vi "监控模板.vi"() -> ()   [LabVIEW 2011]
panel:
  in  "监控":enum32{"RF", "TIME"}(tab)
  out "b 1":bool
  out "b 2":bool
  out "b 3":bool
  out "b 4":bool
  out "b 5":bool
  out "b 6":bool
  out "b 7":bool
  out "b 8":bool
  out "b 9":bool
  out "b 10":bool
  out "b 11":bool
  out "b 12":bool
  out "b 13":bool
  out "b 14":bool
  out "b 15":bool
  out "b 16":bool
  out "b 17":bool
  out "b 18":bool
  out "b 19":bool
  out "b 20":bool
  out "b 21":bool
  out "b 22":bool
  out "b 23":bool
  out "b 24":bool
  out "b 25":bool
  out "b 26":bool
  out "b 27":bool
  out "b 28":bool
  out "b 29":bool
  out "b 30":bool
  out "b 31":bool
  out "b 32":bool
  out "S 1":string
  out "S 2":string
  out "S 3":string
  out "S 4":string
  out "S 5":string
  out "S 6":string
  out "S 7":string
  out "S 8":string
  out "S 9":string
  out "S 10":string
  out "S 11":string
  out "S 12":string
  out "S 13":string
  out "S 14":string
  out "S 15":string
  out "S 16":string
  out "S 17":string
  out "S 18":string
  out "S 19":string
  out "S 20":string
  out "S 21":string
  out "S 22":string
  out "S 23":string
  out "S 24":string
  out "S 25":string
  out "S 26":string
  out "S 27":string
  out "S 28":string
  out "S 29":string
  out "S 30":string
  out "S 31":string
  out "S 32":string
  out "b 33":bool
  out "b 41":bool
  out "b 49":bool
  out "b 57":bool
  out "S 33":string
  out "S 41":string
  out "S 49":string
  out "S 57":string
  out "a 9":bool
  out "b 34":bool
  out "b 42":bool
  out "b 50":bool
  out "b 58":bool
  out "S 34":string
  out "S 42":string
  out "S 50":string
  out "S 58":string
  out "a 10":bool
  out "b 35":bool
  out "b 43":bool
  out "b 51":bool
  out "b 59":bool
  out "S 35":string
  out "S 43":string
  out "S 51":string
  out "S 59":string
  out "a 11":bool
  out "b 36":bool
  out "b 44":bool
  out "b 52":bool
  out "b 60":bool
  out "S 36":string
  out "S 44":string
  out "S 52":string
  out "S 60":string
  out "a 12":bool
  out "b 37":bool
  out "b 45":bool
  out "b 53":bool
  out "b 61":bool
  out "S 37":string
  out "S 45":string
  out "S 53":string
  out "S 61":string
  out "a 13":bool
  out "b 38":bool
  out "b 46":bool
  out "b 54":bool
  out "b 62":bool
  out "S 38":string
  out "S 46":string
  out "S 54":string
  out "S 62":string
  out "a 14":bool
  out "b 39":bool
  out "b 47":bool
  out "b 55":bool
  out "b 63":bool
  out "S 39":string
  out "S 47":string
  out "S 55":string
  out "S 63":string
  out "a 15":bool
  out "b 40":bool
  out "b 48":bool
  out "b 56":bool
  out "b 64":bool
  out "S 40":string
  out "S 48":string
  out "S 56":string
  out "S 64":string
  out "a 16":bool
  out "A 9":bool
  out "A 16":bool
  out "A 15":bool
  out "A 14":bool
  out "A 13":bool
  out "A 12":bool
  out "A 11":bool
  out "A 10":bool
  out "A 1":bool
  out "a 1":bool
  out "a 2":bool
  out "A 2":bool
  out "a 3":bool
  out "A 3":bool
  out "a 4":bool
  out "A 4":bool
  out "a 5":bool
  out "A 5":bool
  out "a 6":bool
  out "A 6":bool
  out "a 7":bool
  out "A 7":bool
  out "a 8":bool
  out "A 8":bool
  out "COM 1":bool
  out "com_1":bool
  out "com_2":bool
  out "COM 2":bool
  out "com_3":bool
  out "COM 3":bool
  out "com_4":bool
  out "COM 4":bool
  out "T 1":bool caption="1"
  out "T 2":bool caption="2"
  out "T 3":bool caption="3"
  out "T 4":bool caption="4"
  out "T 5":bool caption="5"
  out "T 6":bool caption="6"
  out "T 7":bool caption="7"
  out "T 8":bool caption="8"
  out "T 9":bool caption="9"
  out "T 10":bool caption="10"
  out "T 11":bool caption="11"
  out "T 12":bool caption="12"
  out "T 13":bool caption="13"
  out "T 14":bool caption="14"
  out "T 15":bool caption="15"
  out "T 16":bool caption="16"
  out "T 17":bool caption="17"
  out "T 18":bool caption="18"
  out "T 19":bool caption="19"
  out "T 20":bool caption="20"
  out "T 21":bool caption="21"
  out "T 22":bool caption="22"
  out "T 23":bool caption="23"
  out "T 24":bool caption="24"
  out "T 25":bool caption="25"
  out "T 26":bool caption="26"
  out "T 27":bool caption="27"
  out "T 28":bool caption="28"
  out "T 29":bool caption="29"
  out "T 30":bool caption="30"
  out "T 31":bool caption="31"
  out "T 32":bool caption="32"
  out "T 33":bool caption="33"
  out "T 34":bool caption="34"
  out "T 35":bool caption="35"
  out "T 36":bool caption="36"
  out "T 37":bool caption="37"
  out "T 38":bool caption="38"
  out "T 39":bool caption="39"
  out "T 40":bool caption="40"
  out "T 41":bool caption="41"
  out "T 42":bool caption="42"
  out "T 43":bool caption="43"
  out "T 44":bool caption="44"
  out "T 45":bool caption="45"
  out "T 46":bool caption="46"
  out "T 47":bool caption="47"
  out "T 48":bool caption="48"
  out "OUT 1":bool
  out "OUT 2":bool
  out "OUT 4":bool
  out "OUT 3":bool
  out "OUT 5":bool
  out "OUT 6":bool
  out "OUT 8":bool
  out "OUT 7":bool
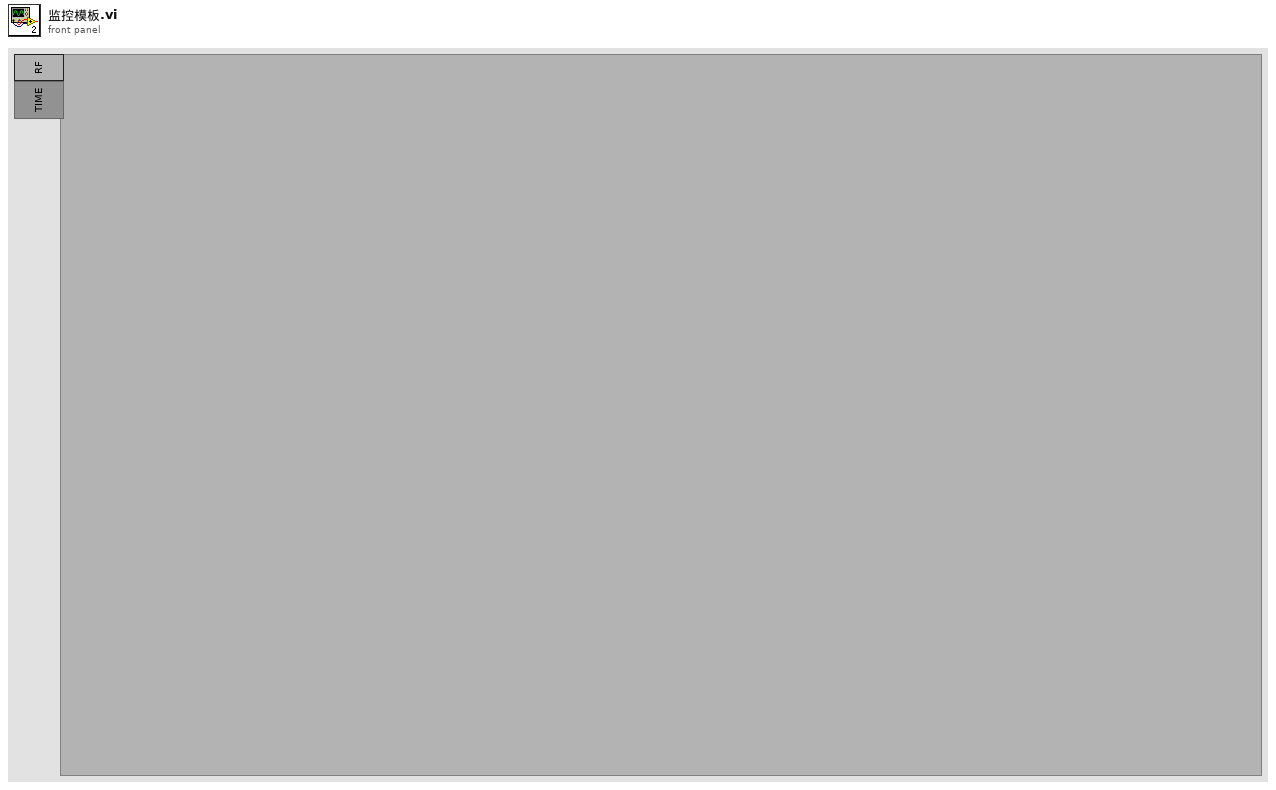
[diagram p1: front panel]
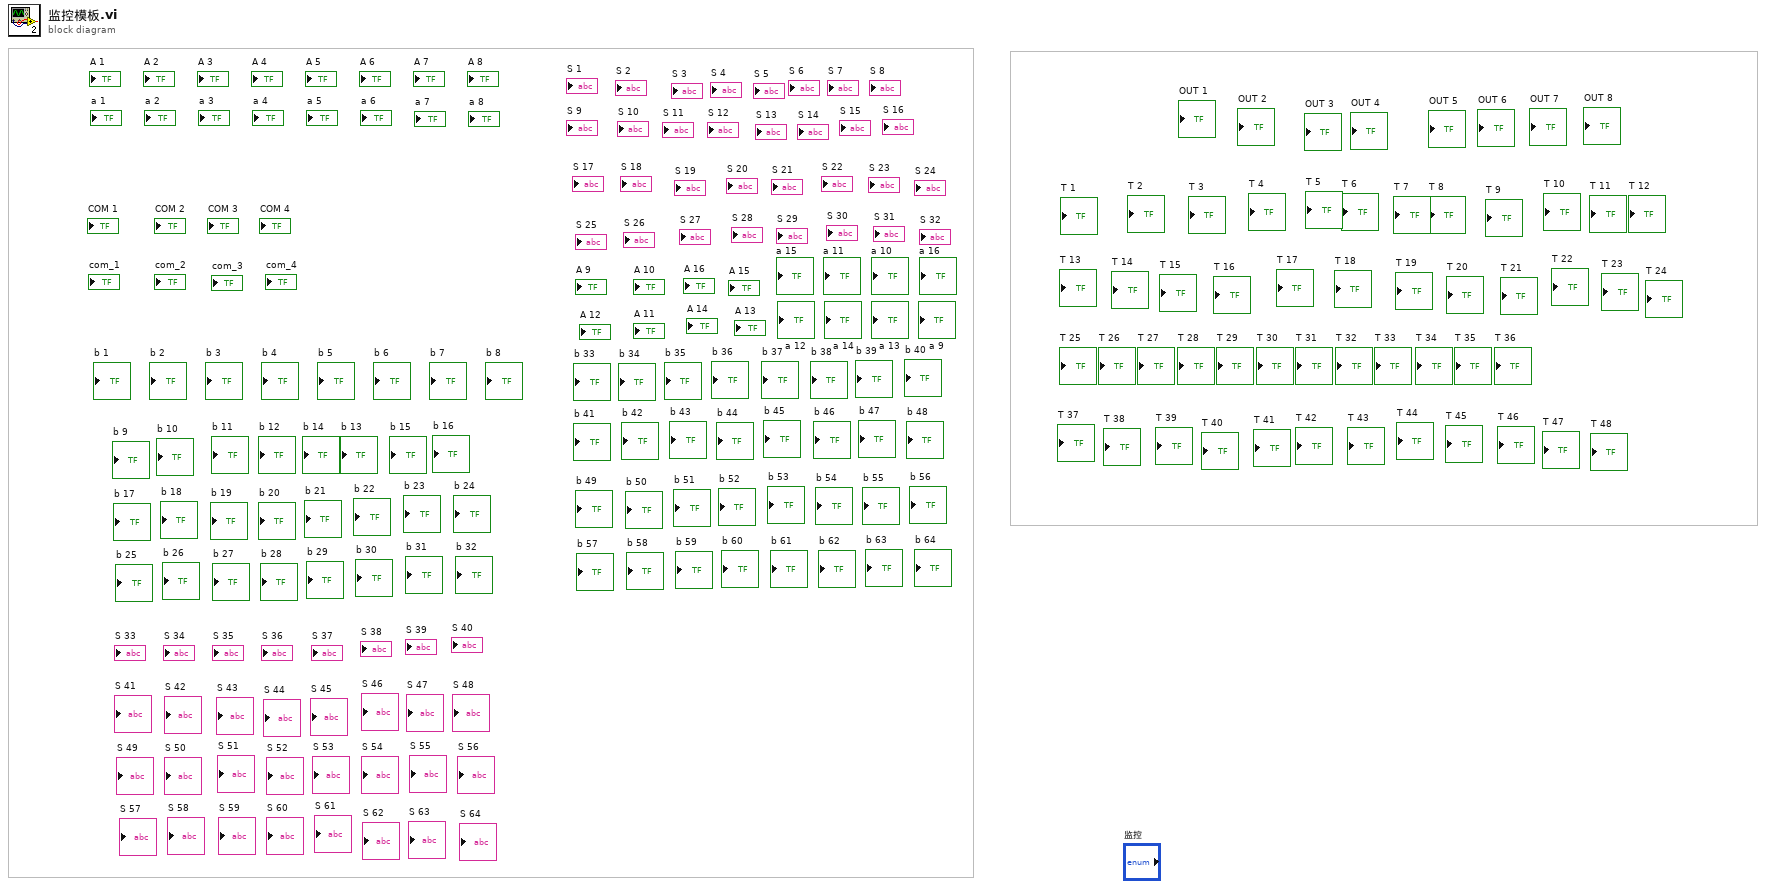
[diagram p0: block diagram]
diagram:
